vi "Set Interface Ref.vi"(8 "error in (no error)":errorcluster, 10 "interface ref":refnum<data-value>, 11 "output_actor in":refnum<class "Output Actor.lvclass">) -> (0 "error out":errorcluster, 3 "output_actor out":refnum<class "Output Actor.lvclass">)   [LabVIEW 2015, in "Output Actor.lvclass"]
uses:
  Output Actor.lvclass
  Output Actor Interface/Output Actor Interface.lvclass
  Output Actor.lvclass/Output Actor.ctl
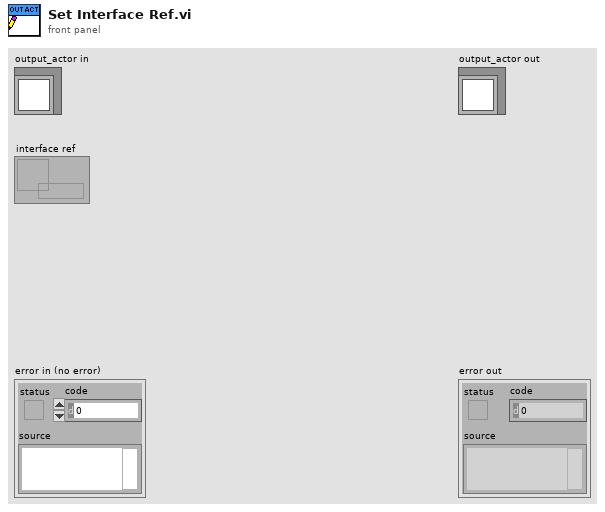
[diagram p1: front panel]
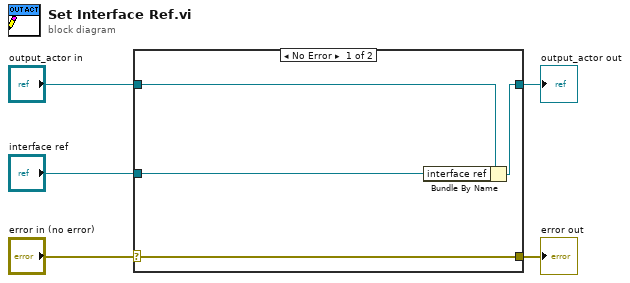
[diagram p0: block diagram]
diagram:
  n1 = case shown="No Error" "error in (no error)" {
    selector: "error in (no error)" -> [w9 w10]
    tunnel: [w9 w10] -> w4
    tunnel: [w7 w11] -> w2
    tunnel: "output_actor in" -> [w8 w11]
    tunnel: "interface ref" -> [w6 _]
    frame No Error {
      n2 = Bundle By Name(cluster=w8, "interface ref"=w6) -> (w7:refnum<class "Output Actor.lvclass">)
    }
    frame Error {
    }
  }
  "error out" <- w4
  "output_actor out" <- w2
